vi "Legend Palette.vi"(4 "Active Plot":i32, 6 "Control Ref Queue":T1, 9 "Window Bounds":T5, 10 "Multiplot Representation In":T2, 11 "2D Error Bar.lvclass in":refnum<class "2D Error Bar.lvclass">) -> (1 "Cancel?":bool, 2 "Multiplot Representation Out":T2, 3 "2D Error Bar.lvclass out":refnum<class "2D Error Bar.lvclass">)   [LabVIEW 2017, in "2D Error Bar.lvclass"]
uses:
  <vilib>/Math Plots/2D Math Plots/2D Error Bar/2D Error Bar/2D Error Bar.lvclass
  <vilib>/Math Plots/2D Math Plots/2D Plot/2D Plot/Typedef/Multiplot Representation.ctl
  <vilib>/Math Plots/2D Math Plots/2D Plot/2D Plot/Typedef/Plot Representation.ctl
  <vilib>/Math Plots/2D Math Plots/2D Plot/2D Plot/Typedef/Range Cluster.ctl
  <vilib>/Math Plots/2D Math Plots/2D Plot/Action String/2DMathPlot Ctrl Act Queue.ctl
  <vilib>/Math Plots/2D Math Plots/2D Plot/Action String/2DMathPlot Ctrl Act Cluster.ctl
  <vilib>/Math Plots/2D Math Plots/2D Plot/Action String/2DMathPlot State Class.ctl
  e:/builds/penguin/labview/branches/2017/dev/dist/vi.lib/Math Plots/2D Math Plots/2D Plot/2D Plot/2D Plot.lvclass
  <vilib>/Utility/miscctls.llb/LVRectTypeDef.ctl
  <vilib>/Math Plots/2D Math Plots/2D Error Bar/2D Error Bar/2D Error Bar.lvclass/2D Error Bar.ctl
  <vilib>/Math Plots/2D Math Plots/2D Plot/2D Plot/2D Plot.lvclass
panel:
  in  "Tab Control":enum32{"Plot Property", "Input & Output"}(tab)
  in  "Fill To":u16(ring) caption="Line width"
  in  "Marker Style":u16(ring) caption="Line style"
  in  "Marker Width":u16(ring) caption="Line width"
  in  "Fill Color":u32(colorbox)
  in  "Fill Style":u16(ring) caption="Line style"
  in  "Point Style":u16(ring) caption="Line width"
  in  "Line Color":u32(colorbox)
  in  "Marker Color":u32(colorbox)
  in  "Marker Size":dbl caption="Error Bar size"
  in  "Cancel":bool
  in  "OK":bool
  in  "Line Style":u16(ring) caption="Line style"
  in  "Line Width":u16(ring) caption="Line width"
  # "Line style"
  # "Line width"
  # "Line color"
  # "Point style"
  # "Fill style"
  # "Fill to"
  # "Point/fill color"
  # "Marker width"
  # "Marker style"
  # "Marker color"
  # "Marker size"
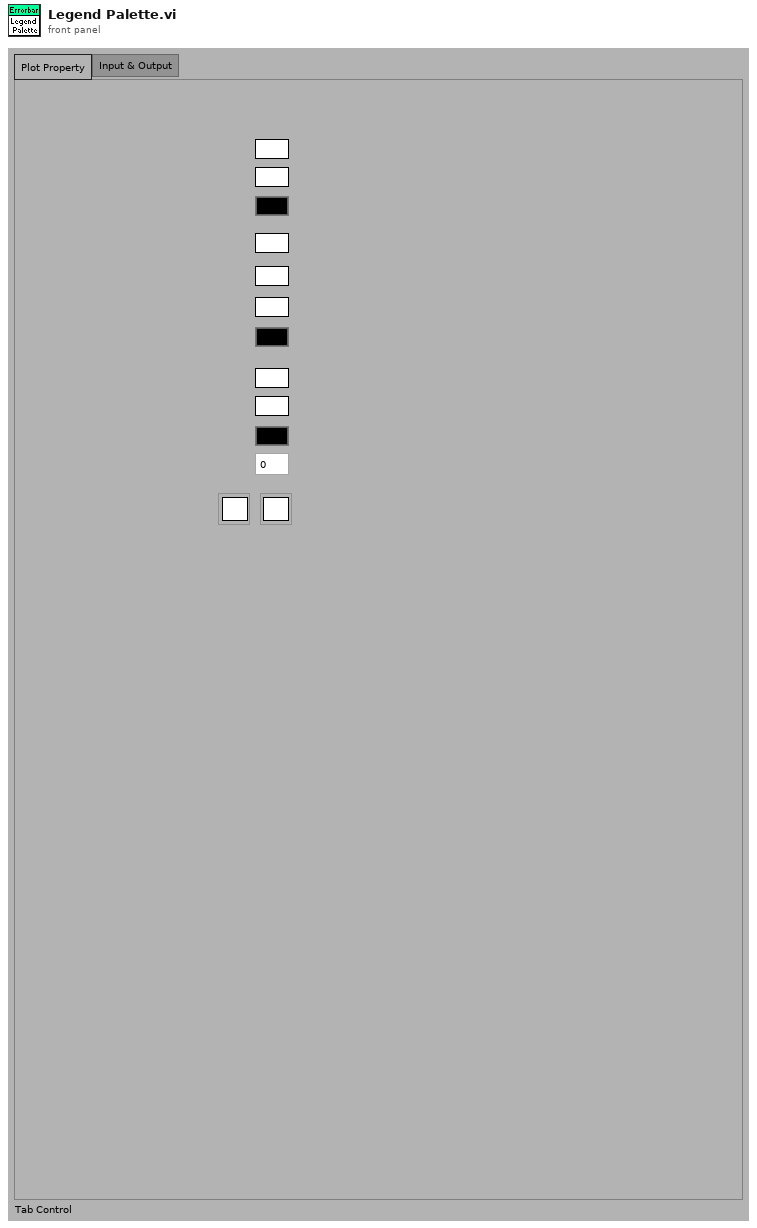
[diagram p1: front panel]
types:
  T1 = typedef "2DMathPlot Ctrl Act Queue.ctl" = refnum<queue>
  T2 = typedef "2D Plot.lvclass/Multiplot Representation.ctl" = cluster{"Plot Representation Array":T3[], "Max Range":T4}
  T3 = typedef "2D Plot.lvclass/Plot Representation.ctl" = cluster{"Plot Range":T4, "Vertex Cluster":cluster{"Vertex X Array":dbl[], "Vertex Y Array":dbl[]}, "Base Cluster":cluster{"Base X Array":dbl[], "Base Y Array":dbl[]}}
  T4 = typedef "2D Plot.lvclass/Range Cluster.ctl" = cluster{"X Range":cluster{"Max X":dbl, "Min X":dbl}, "Y Range":cluster{"Max Y":dbl, "Min Y":dbl}}
  T5 = typedef "LVRectTypeDef.ctl" = cluster{"Left":i16, "Top":i16, "Right":i16, "Bottom":i16}
  T6 = typedef "2DMathPlot Ctrl Act Cluster.ctl" = cluster{"Plot Area Ref":refnum<vi>, "Z Axis Ref":refnum<vi>, "Legend Ref":refnum<vi>, "XControl Ref":refnum<vi>, "Facade Ref":refnum<vi>, "Display State Change Class":T7}
  T7 = typedef "2DMathPlot State Class.ctl" = enum16{"Update All (Undo)", "Update General", "Update Appearance", "Update Format", "Update Scale", "Update Marker", "Update Cursor", "None"}
  T8 = typedef "2D Plot.lvclass/Plot Property Array.ctl" = T9[]
  T9 = typedef "2D Plot.lvclass/Plot Property.ctl" = cluster{"Bar Plot Style":u8, "DigitalLineStyle":u8, "TransitionLocation":u8, "Transition Type":u8, "Fill To":i16, "Fill/Pt. Color":u32, "Label Style":u8, "Line Style":u8, "Line Width":u8, "Plot Color":u32, "Plot Interpolation":u8, "Plot Name":string, "Point Style":u8, "Visible?":bool, "XScaleIdx":u32, "YScaleIdx":u32}
  T10 = typedef "2D Error Bar.lvclass/2D Error Bar Property Array.ctl" = T11[]
  T11 = typedef "2D Error Bar.lvclass/2D Error Bar Property.ctl" = cluster{"Marker Size":dbl, "Marker Line Style":u8, "Marker Line Width":u8, "Marker Color":u32, "Error Bar Interpolation":enum16{"Show Point", "Show Line", "Show Bar"}, "Error Mode":enum16{"Show Y Error", "Show X Error", "Show Both Error"}}
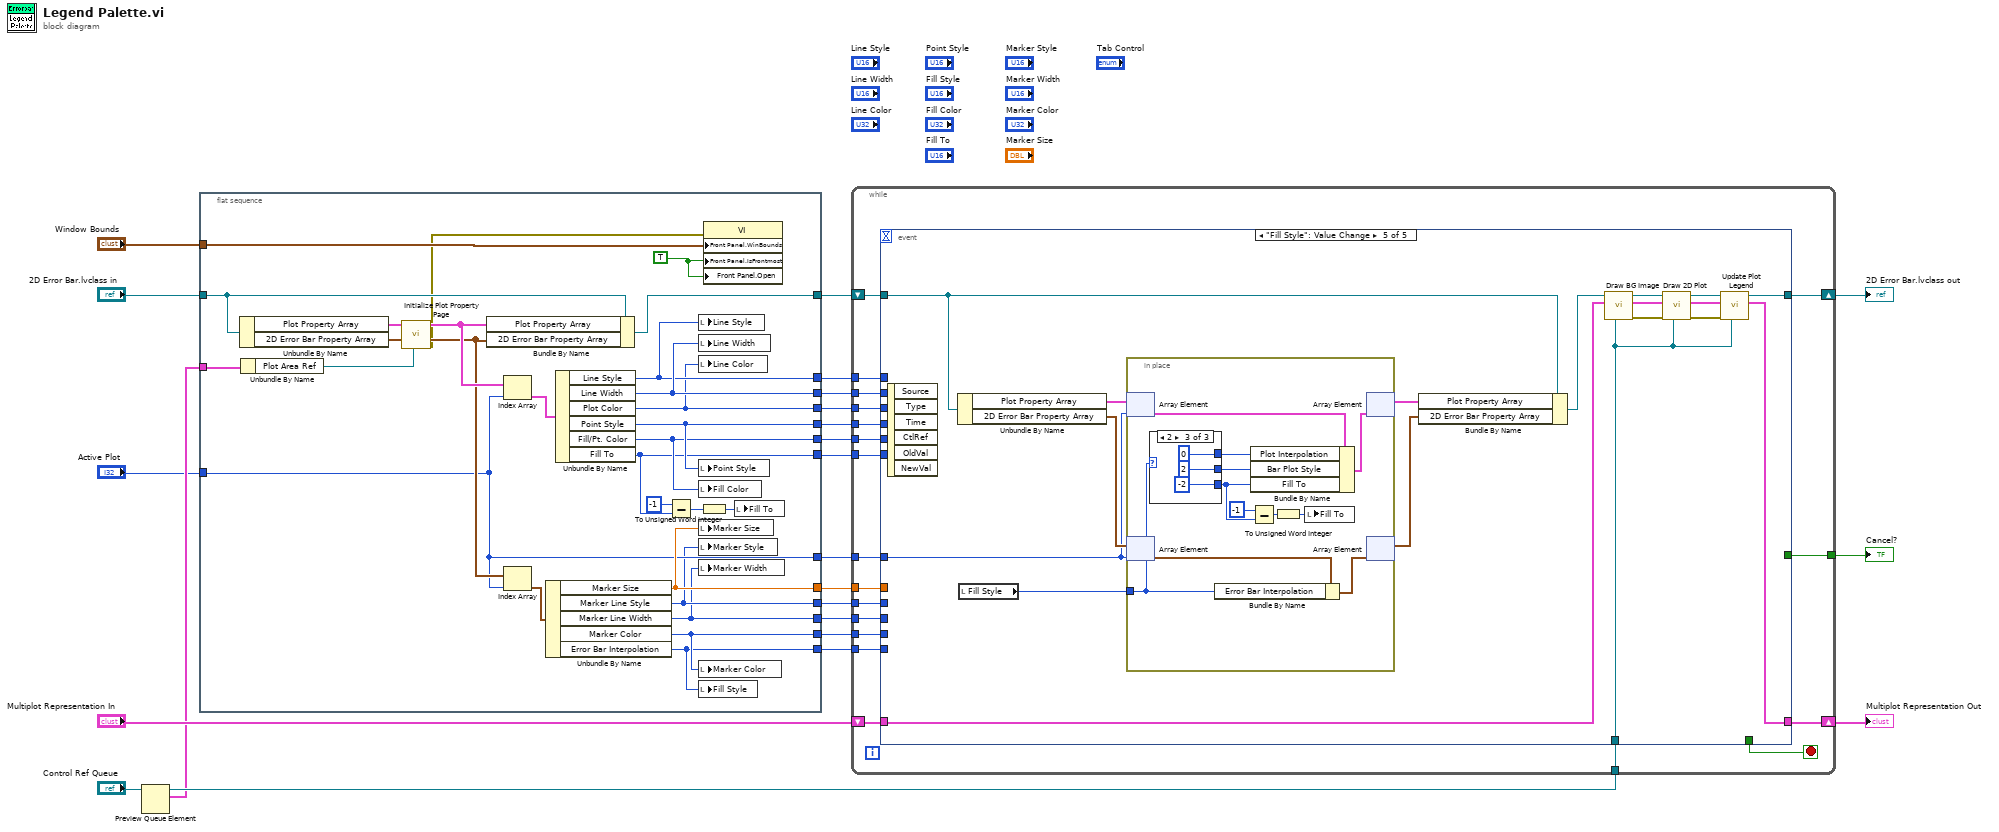
[diagram p0: block diagram]
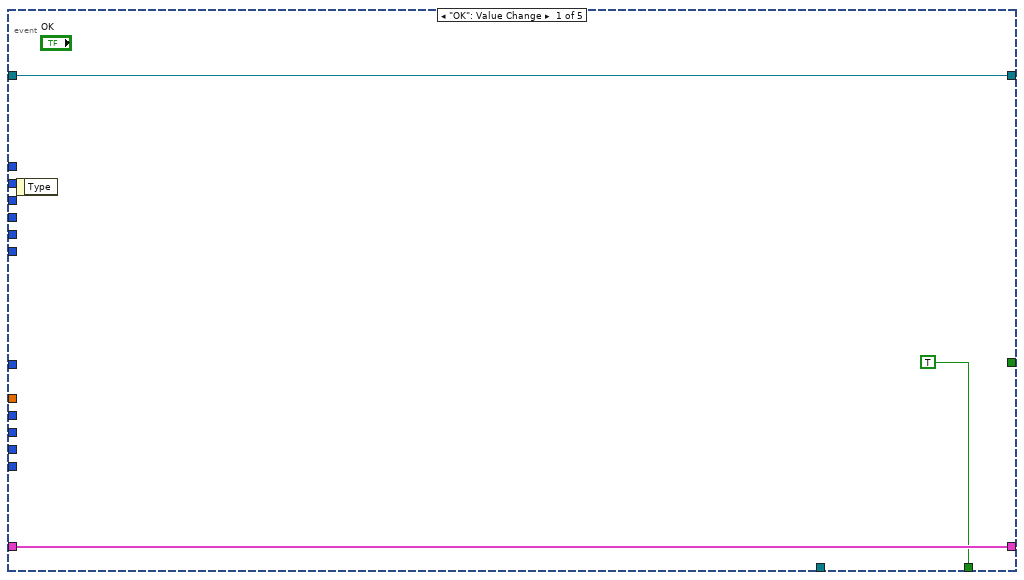
[diagram p2: hidden frame]
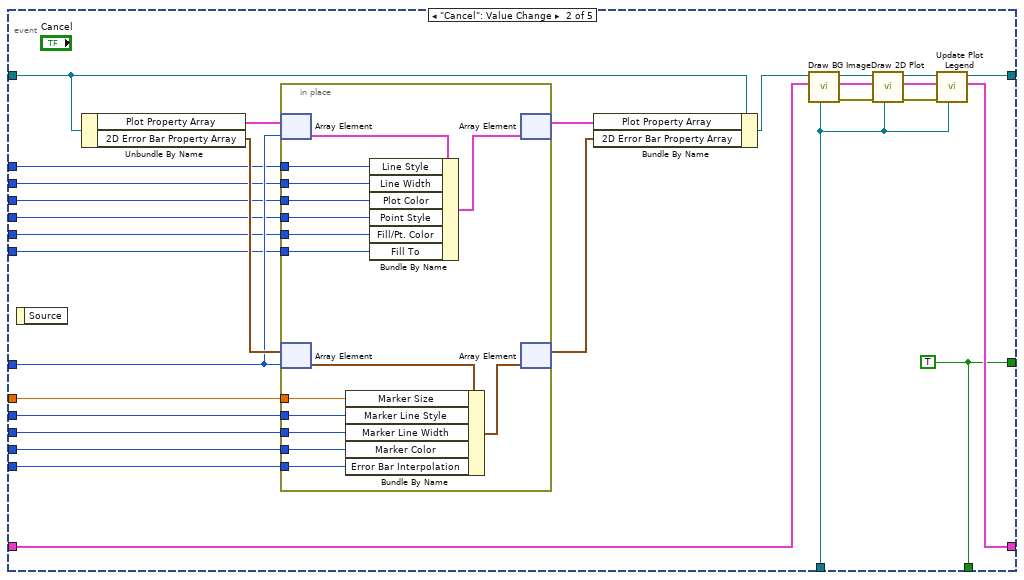
[diagram p3: hidden frame]
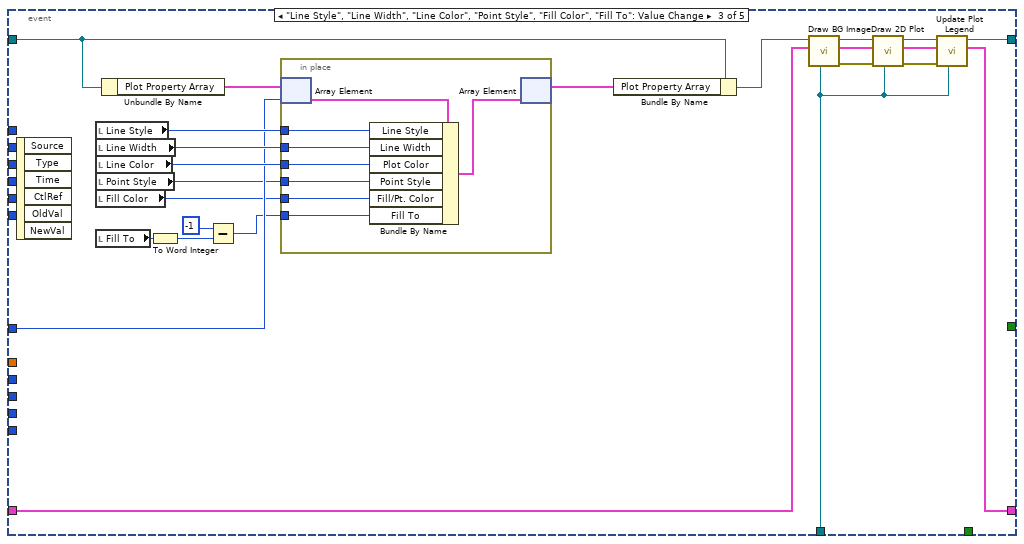
[diagram p4: hidden frame]
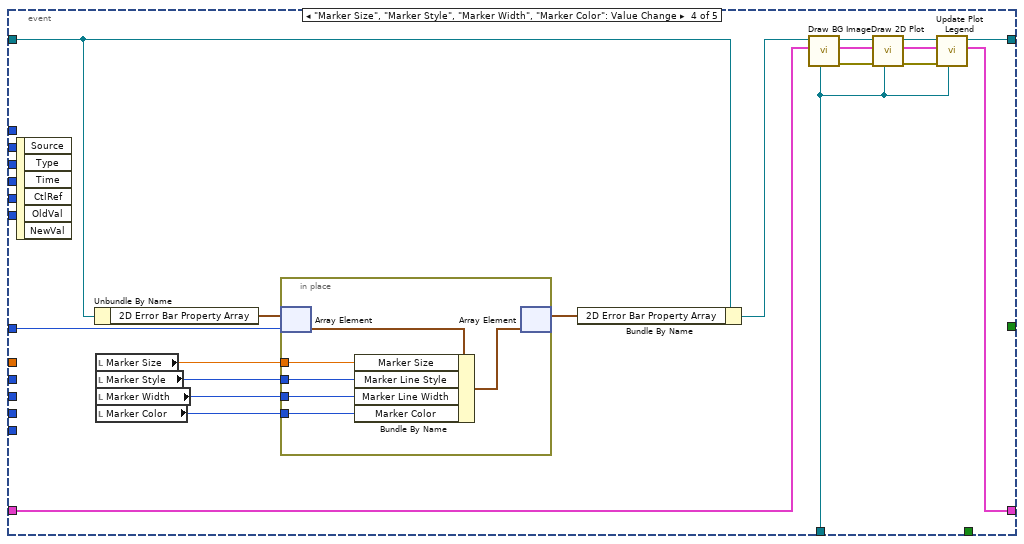
[diagram p5: hidden frame]
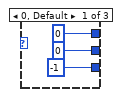
[diagram p6: hidden frame]
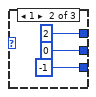
[diagram p7: hidden frame]
diagram:
  n1 = Preview Queue Element(queue="Control Ref Queue") -> (queue out=w17:T1, element=w16:T6)  [unwired: 1 in, 3 out]
  n2 = flat-sequence {
    tunnel: "2D Error Bar.lvclass in" -> [w40]
    tunnel: [w39] -> w21
    tunnel: [w35] -> w11
    tunnel: w16 -> [w49]
    tunnel: [w47] -> w15
    tunnel: [w34] -> w14
    tunnel: [w46] -> w13
    tunnel: [w45] -> w12
    tunnel: "Window Bounds" -> [w37]
    tunnel: "Active Plot" -> [w35]
    tunnel: [w33] -> w7
    tunnel: [w32] -> w6
    tunnel: [w26] -> w5
    tunnel: [w31] -> w4
    tunnel: [w30] -> w3
    tunnel: [w29] -> w2
    tunnel: [w28] -> w1
    frame #0 {
      w48 = TRUE ("Front Panel Window:Is Frontmost")
      n3 = Unbundle By Name(w40) -> ("Plot Property Array"=w44:T8, "2D Error Bar Property Array"=w43:T10)
      n4 = Unbundle By Name(w49) -> ("Plot Area Ref"=w38:refnum<vi>)
      n5 = call <vilib>:"Initialize Plot Property Page.vi"("Plot Area Ref"=w38, "2D Error Bar Array In"=w43, "Plot Property Array In"=w44) -> ("error out"=w36:errorcluster, "2D Error Bar Array Out"=w41:T10, "Plot Property Array Out"=w42:T8)  [unwired: 2 in, 4 out]
      n6 = Bundle By Name(cluster=w40, "Plot Property Array"=w42, "2D Error Bar Property Array"=w41) -> (w39:refnum<class "2D Error Bar.lvclass">)
      n7 = Index Array(array=w42, index=w35) -> (element=w51:T9)
      n8 = Index Array(array=w41, index=w35) -> (element=w50:T11)
      n9 = Unbundle By Name(w50) -> ("Marker Size"=w47:dbl, "Marker Line Style"=w31:u8, "Marker Line Width"=w30:u8, "Marker Color"=w29:u32, "Error Bar Interpolation"=w28:enum16{"Show Point", "Show Line", "Show Bar"})
      n10 = Unbundle By Name(w51) -> ("Line Style"=w45:u8, "Line Width"=w46:u8, "Plot Color"=w34:u32, "Point Style"=w33:u8, "Fill/Pt. Color"=w32:u32, "Fill To"=w26:i16)
      n11 = Subtract(x=i16 -1, y=w26) -> (x-y=w25:i16)
      n12 = local write "Line Style"(w45) -> ()
      n13 = local write "Line Width"(w46) -> ()
      n14 = local write "Line Color"(w34) -> ()
      n15 = local write "Point Style"(w33) -> ()
      n16 = local write "Fill Color"(w32) -> ()
      n17 = local write "Marker Size"(w47) -> ()
      n18 = local write "Marker Style"(w31) -> ()
      n19 = local write "Marker Width"(w30) -> ()
      n20 = local write "Marker Color"(w29) -> ()
      n21 = local write "Fill Style"(w28) -> ()
      n22 = To Unsigned Word Integer(number=w25) -> (unsigned 16bit integer=w24:u16)
      n23 = property class="VI"(error in=w36, "Front Panel.WinBounds"=w37, "Front Panel.IsFrontmost"=w48, "Front Panel.Open"=w48) -> ()  [unwired: 1 in, 2 out]
      n24 = local write "Fill To"(w24) -> ()
    }
  }
  n25 = while {
    shift-right: [w69] -> w23
    shift-left: w21 -> [w70]
    shift-right: [w67] -> w19
    shift-left: "Multiplot Representation In" -> [w68]
    tunnel: w17 -> [w66]
    tunnel: w11 -> [w65]
    tunnel: w15 -> [w63]
    tunnel: w14 -> [w62]
    tunnel: w13 -> [w61]
    tunnel: w12 -> [w60]
    tunnel: [w59] -> w10
    tunnel: w7 -> [w58]
    tunnel: w6 -> [w57]
    tunnel: w5 -> [w56]
    tunnel: w4 -> [w55]
    tunnel: w3 -> [w54]
    tunnel: w2 -> [w53]
    tunnel: w1 -> [w52]
    stop <- w64 stop-if-true
    n26 = event shown="[4] \"Fill Style\": Value Change" {
      selector: _ -> [_ _ _ _ _]
      dyn-events: _ -> [_ _ _ _ _]
      timeout: _ -> [_ _ _ _ _]
      tunnel: w70 -> [w73 w97 w140 w167 w191]
      tunnel: [w73 w90 w132 w162 w187] -> w69
      tunnel: w68 -> [w72 w96 w134 w163 w188]
      tunnel: [w72 w89 w131 w161 w186] -> w67
      tunnel: w66 -> [_ w82 w124 w154 w179]
      tunnel: w65 -> [_ w95 w133 w150 w176]
      tunnel: [TRUE w81 _ _ _] -> w64
      tunnel: w63 -> [_ w94 _ _ _]
      tunnel: w62 -> [_ w93 _ _ _]
      tunnel: w61 -> [_ w92 _ _ _]
      tunnel: w60 -> [_ w91 _ _ _]
      tunnel: [_ w81 _ _ _] -> w59
      tunnel: w58 -> [_ w76 _ _ _]
      tunnel: w57 -> [_ w75 _ _ _]
      tunnel: w56 -> [_ w74 _ _ _]
      tunnel: w55 -> [_ w80 _ _ _]
      tunnel: w54 -> [_ w79 _ _ _]
      tunnel: w53 -> [_ w78 _ _ _]
      tunnel: w52 -> [_ w77 _ _ _]
      event "OK": Value Change {
        n27 = event-data() -> ()  [unwired: 2 out]
      }
      event "Cancel": Value Change {
        w81 = TRUE
        n28 = event-data() -> ()  [unwired: 2 out]
        n29 = Unbundle By Name(w97) -> ("Plot Property Array"=w102:T8, "2D Error Bar Property Array"=w101:T10)
        n30 = in-place {
          in-place-border: w94 -> [w113]
          in-place-border: w91 -> [w112]
          in-place-border: w92 -> [w111]
          in-place-border: w93 -> [w110]
          in-place-border: w80 -> [w109]
          in-place-border: w79 -> [w108]
          in-place-border: w78 -> [w107]
          in-place-border: w77 -> [w106]
          in-place-border: w76 -> [w105]
          in-place-border: w75 -> [w104]
          in-place-border: w74 -> [w103]
          n31 = in-place-array #1(w102, w95) -> (w117:T9)
          n32 = in-place-array #2(w101, w95) -> (w116:T11)
          n33 = Bundle By Name(cluster=w116, "Marker Size"=w113, "Marker Line Style"=w109, "Marker Line Width"=w108, "Marker Color"=w107, "Error Bar Interpolation"=w106) -> (w115:T11)
          n34 = Bundle By Name(cluster=w117, "Line Style"=w112, "Line Width"=w111, "Plot Color"=w110, "Point Style"=w105, "Fill/Pt. Color"=w104, "Fill To"=w103) -> (w114:T9)
          n35 = in-place-array #1(w114) -> (w100:T8)  [unwired: 1 out]
          n36 = in-place-array #2(w115) -> (w99:T10)  [unwired: 1 out]
        }
        n37 = Bundle By Name(cluster=w97, "Plot Property Array"=w100, "2D Error Bar Property Array"=w99) -> (w98:refnum<class "2D Error Bar.lvclass">)
        n38 = call-dynamic "Draw BG Image.vi"("Control Ref Queue"=w82, "Multiplot Representation In"=w96, "2D Error Bar.lvclass in"=w98) -> ("error out"=w88:errorcluster, "Multiplot Representation Out"=w87:T2, "2D Error Bar.lvclass out"=w86:refnum<class "2D Error Bar.lvclass">)  [unwired: 1 in, 5 out]
        n39 = call-dynamic "Draw 2D Plot.vi"("Control Ref Queue"=w82, "error in (no error)"=w88, "Multiplot Representation In"=w87, "2D Error Bar.lvclass in"=w86) -> ("error out"=w83:errorcluster, "Multiplot Representation Out"=w84:T2, "2D Error Bar.lvclass out"=w85:refnum<class "2D Error Bar.lvclass">)  [unwired: 5 out]
        n40 = call <vilib>:"Update Plot Legend.vi"("Control Ref Queue"=w82, "error in (no error)"=w83, "Multiplot Representation In"=w84, "2D Plot in"=w85) -> ("Multiplot Representation Out"=w89:T2, "2D Plot out"=w90:refnum<class "2D Error Bar.lvclass">)  [unwired: 6 out]
      }
      event "Line Style", "Line Width", "Line Color", "Point Style", "Fill Color", "Fill To": Value Change {
        n41 = event-data() -> ()  [unwired: 7 out]
        n42 = local read "Line Style"() -> (w138:u16)
        n43 = local read "Line Width"() -> (w137:u16)
        n44 = local read "Line Color"() -> (w136:u32)
        n45 = local read "Point Style"() -> (w123:u16)
        n46 = local read "Fill Color"() -> (w122:u32)
        n47 = local read "Fill To"() -> (w120:u16)
        n48 = Unbundle By Name(w140) -> ("Plot Property Array"=w141:T8)
        n49 = To Word Integer(number=w120) -> (16bit integer=w118:i16)
        n50 = Subtract(x=i16 -1, y=w118) -> (x-y=w121:i16)
        n51 = in-place {
          in-place-border: w138 -> [w147]
          in-place-border: w137 -> [w146]
          in-place-border: w136 -> [w145]
          in-place-border: w123 -> [w144]
          in-place-border: w122 -> [w143]
          in-place-border: w121 -> [w142]
          n52 = in-place-array #3(w141, w133) -> (w149:T9)
          n53 = Bundle By Name(cluster=w149, "Line Style"=w147, "Line Width"=w146, "Plot Color"=w145, "Point Style"=w144, "Fill/Pt. Color"=w143, "Fill To"=w142) -> (w148:T9)
          n54 = in-place-array #3(w148) -> (w139:T8)  [unwired: 1 out]
        }
        n55 = Bundle By Name(cluster=w140, "Plot Property Array"=w139) -> (w135:refnum<class "2D Error Bar.lvclass">)
        n56 = call-dynamic "Draw BG Image.vi"("Control Ref Queue"=w124, "Multiplot Representation In"=w134, "2D Error Bar.lvclass in"=w135) -> ("error out"=w130:errorcluster, "Multiplot Representation Out"=w129:T2, "2D Error Bar.lvclass out"=w128:refnum<class "2D Error Bar.lvclass">)  [unwired: 1 in, 5 out]
        n57 = call-dynamic "Draw 2D Plot.vi"("Control Ref Queue"=w124, "error in (no error)"=w130, "Multiplot Representation In"=w129, "2D Error Bar.lvclass in"=w128) -> ("error out"=w125:errorcluster, "Multiplot Representation Out"=w126:T2, "2D Error Bar.lvclass out"=w127:refnum<class "2D Error Bar.lvclass">)  [unwired: 5 out]
        n58 = call <vilib>:"Update Plot Legend.vi"("Control Ref Queue"=w124, "error in (no error)"=w125, "Multiplot Representation In"=w126, "2D Plot in"=w127) -> ("Multiplot Representation Out"=w131:T2, "2D Plot out"=w132:refnum<class "2D Error Bar.lvclass">)  [unwired: 6 out]
      }
      event "Marker Size", "Marker Style", "Marker Width", "Marker Color": Value Change {
        n59 = event-data() -> ()  [unwired: 7 out]
        n60 = Unbundle By Name(w167) -> ("2D Error Bar Property Array"=w168:T10)
        n61 = local read "Marker Size"() -> (w165:dbl)
        n62 = local read "Marker Style"() -> (w153:u16)
        n63 = local read "Marker Width"() -> (w152:u16)
        n64 = local read "Marker Color"() -> (w151:u32)
        n65 = in-place {
          in-place-border: w165 -> [w172]
          in-place-border: w153 -> [w171]
          in-place-border: w152 -> [w170]
          in-place-border: w151 -> [w169]
          n66 = in-place-array #4(w168, w150) -> (w174:T11)
          n67 = Bundle By Name(cluster=w174, "Marker Size"=w172, "Marker Line Style"=w171, "Marker Line Width"=w170, "Marker Color"=w169) -> (w173:T11)
          n68 = in-place-array #4(w173) -> (w166:T10)  [unwired: 1 out]
        }
        n69 = Bundle By Name(cluster=w167, "2D Error Bar Property Array"=w166) -> (w164:refnum<class "2D Error Bar.lvclass">)
        n70 = call-dynamic "Draw BG Image.vi"("Control Ref Queue"=w154, "Multiplot Representation In"=w163, "2D Error Bar.lvclass in"=w164) -> ("error out"=w160:errorcluster, "Multiplot Representation Out"=w159:T2, "2D Error Bar.lvclass out"=w158:refnum<class "2D Error Bar.lvclass">)  [unwired: 1 in, 5 out]
        n71 = call-dynamic "Draw 2D Plot.vi"("Control Ref Queue"=w154, "error in (no error)"=w160, "Multiplot Representation In"=w159, "2D Error Bar.lvclass in"=w158) -> ("error out"=w155:errorcluster, "Multiplot Representation Out"=w156:T2, "2D Error Bar.lvclass out"=w157:refnum<class "2D Error Bar.lvclass">)  [unwired: 5 out]
        n72 = call <vilib>:"Update Plot Legend.vi"("Control Ref Queue"=w154, "error in (no error)"=w155, "Multiplot Representation In"=w156, "2D Plot in"=w157) -> ("Multiplot Representation Out"=w161:T2, "2D Plot out"=w162:refnum<class "2D Error Bar.lvclass">)  [unwired: 6 out]
      }
      event "Fill Style": Value Change {
        n73 = event-data() -> ()  [unwired: 7 out]
        n74 = Unbundle By Name(w191) -> ("Plot Property Array"=w178:T8, "2D Error Bar Property Array"=w192:T10)
        n75 = local read "Fill Style"() -> (w175:u16)
        n76 = in-place {
          in-place-border: w175 -> [w199]
          n77 = in-place-array #5(w178, w176) -> (w201:T9)
          n78 = in-place-array #6(w192, w176) -> (w203:T11)
          n79 = case shown="2" w199 {
            tunnel: [u8 0 ("Plot Interpolation") u8 2 ("Plot Interpolation") u8 0 ("Plot Interpolation")] -> w197
            tunnel: [u8 0 ("Plot Interpolation") u8 0 ("Plot Interpolation") u8 2 ("Plot Interpolation")] -> w198
            tunnel: [i16 -1 ("Fill To") i16 -1 ("Fill To") i16 -2 ("Fill To")] -> w194
            frame 0, Default {
            }
            frame 1 {
            }
            frame 2 {
            }
          }
          n80 = Bundle By Name(cluster=w203, "Error Bar Interpolation"=w199) -> (w202:T11)
          n81 = Bundle By Name(cluster=w201, "Plot Interpolation"=w197, "Bar Plot Style"=w198, "Fill To"=w194) -> (w200:T9)
          n82 = Subtract(x=i16 -1, y=w194) -> (x-y=w196:i16)
          n83 = To Unsigned Word Integer(number=w196) -> (unsigned 16bit integer=w193:u16)
          n84 = local write "Fill To"(w193) -> ()
          n85 = in-place-array #5(w200) -> (w177:T8)  [unwired: 1 out]
          n86 = in-place-array #6(w202) -> (w190:T10)  [unwired: 1 out]
        }
        n87 = Bundle By Name(cluster=w191, "Plot Property Array"=w177, "2D Error Bar Property Array"=w190) -> (w189:refnum<class "2D Error Bar.lvclass">)
        n88 = call-dynamic "Draw BG Image.vi"("Control Ref Queue"=w179, "Multiplot Representation In"=w188, "2D Error Bar.lvclass in"=w189) -> ("error out"=w185:errorcluster, "Multiplot Representation Out"=w184:T2, "2D Error Bar.lvclass out"=w183:refnum<class "2D Error Bar.lvclass">)  [unwired: 1 in, 5 out]
        n89 = call-dynamic "Draw 2D Plot.vi"("Control Ref Queue"=w179, "error in (no error)"=w185, "Multiplot Representation In"=w184, "2D Error Bar.lvclass in"=w183) -> ("error out"=w180:errorcluster, "Multiplot Representation Out"=w181:T2, "2D Error Bar.lvclass out"=w182:refnum<class "2D Error Bar.lvclass">)  [unwired: 5 out]
        n90 = call <vilib>:"Update Plot Legend.vi"("Control Ref Queue"=w179, "error in (no error)"=w180, "Multiplot Representation In"=w181, "2D Plot in"=w182) -> ("Multiplot Representation Out"=w186:T2, "2D Plot out"=w187:refnum<class "2D Error Bar.lvclass">)  [unwired: 6 out]
      }
    }
  }
  "2D Error Bar.lvclass out" <- w23
  "Multiplot Representation Out" <- w19
  "Cancel?" <- w10
